vi "FGV_AO_WF.vi"(3 "error in 2":errorcluster, 4 "AO WF 3":waveform(dbl)[](graph), 5 "Action 2":T1) -> (0 "error out 2":errorcluster, 1 "AO WF 2":waveform(dbl)[](graph))   [LabVIEW 2025]
uses:
  Controls/TypeDef_FGV.ctl
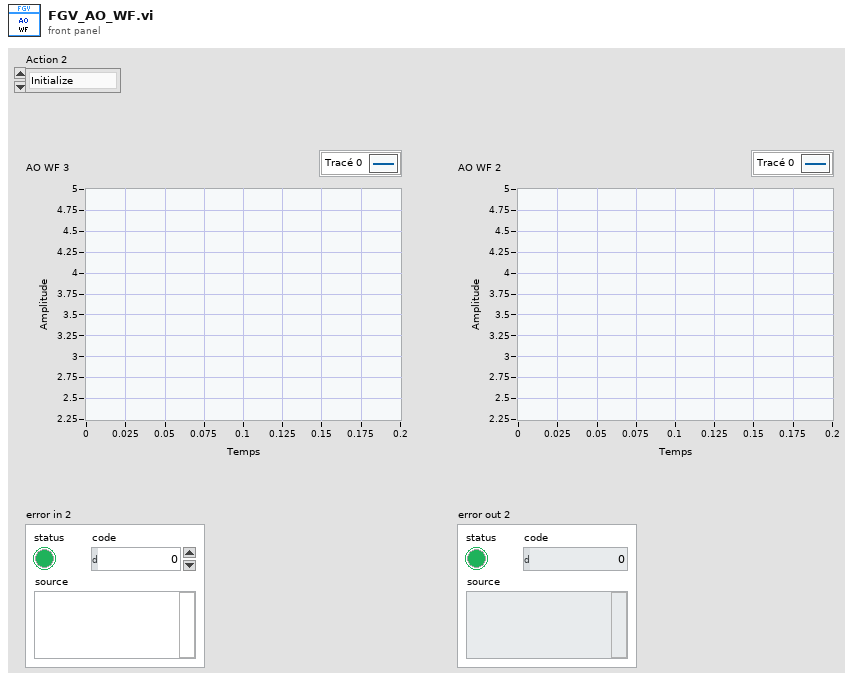
[diagram p1: front panel]
types:
  T1 = typedef "TypeDef_FGV.ctl" = enum16{"Initialize", "Write", "Read"}
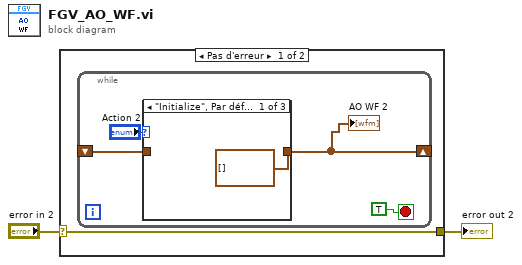
[diagram p0: block diagram]
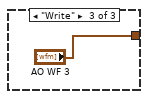
[diagram p3: hidden frame]
diagram:
  n1 = case shown="Pas d'erreur" "error in 2" {
    selector: "error in 2" -> [w3 w11]
    tunnel: [w3 w11] -> w2
    frame No Error {
      n2 = while {
        shift-right: [w4] -> _
        shift-left: _ -> [w5]
        stop <- TRUE stop-if-true
        n3 = case shown="\"Initialize\", Par défaut" "Action 2" {
          tunnel: w5 -> [_ w9 _]
          tunnel: [waveform(dbl)[] [] ("AO WF") w9 "AO WF 3"] -> w4
          frame "Initialize", Default {
          }
          frame "Read" {
          }
          frame "Write" {
          }
        }
        "AO WF 2" <- w4
      }
    }
    frame Error {
    }
  }
  "error out 2" <- w2
